vi "FPGAtdcControlTest.vi"() -> ()   [LabVIEW 2017]
uses:
  <vilib>/FPGAPlugInAG/PXI-7842R/niLvFpga_Open_PXI-7842R.vi
  <vilib>/rvi/interface/common/dynamic/niFpgaDynamicAddResources.vi
  <vilib>/rvi/interface/common/niFpgaWaitOnOcc.vi
  <vilib>/Utility/error.llb/Error Cluster From Error Code.vi
  <vilib>/rvi/errors/niLvFpgaAdjustHostInterfaceError.vi
  <vilib>/rvi/interface/nirviOpenFPGA/nirviOpenFPGA.xnode
  FPGA Bitfiles/Jarvis_FPGATargetMacro_281119simpleTDC_akCax+JGGYk.lvbitx
  <vilib>/rvi/interface/nirviMethod/nirviMethod.xnode
  <vilib>/rvi/interface/nirviReadWriteControl/nirviReadWriteControl.xnode
  NiFpgaLv.dll
  <vilib>/rvi/interface/Simulation/niFpgaSimulationCallBeginRW.vi
  <vilib>/rvi/errors/niLvFpgaMergeErrorWithErrorCode.vi
  <vilib>/FPGAPlugInAG/Dynamic/niLvFpga_ConfigureFifo_Dynamic.vi
  <vilib>/FPGAPlugInAG/Dynamic/niLvFpga_ReadFifo_Dynamic.vi
panel:
  out "error out":errorcluster
  out "Waveform Chart":u32[](graph)
  out "N acquired":i32
  out "Array":i32[](array[numeric])
  out "Histogram":dynamicdata(graph)
  out "tau":i16
  out "new data":bool
  in  "stop":bool
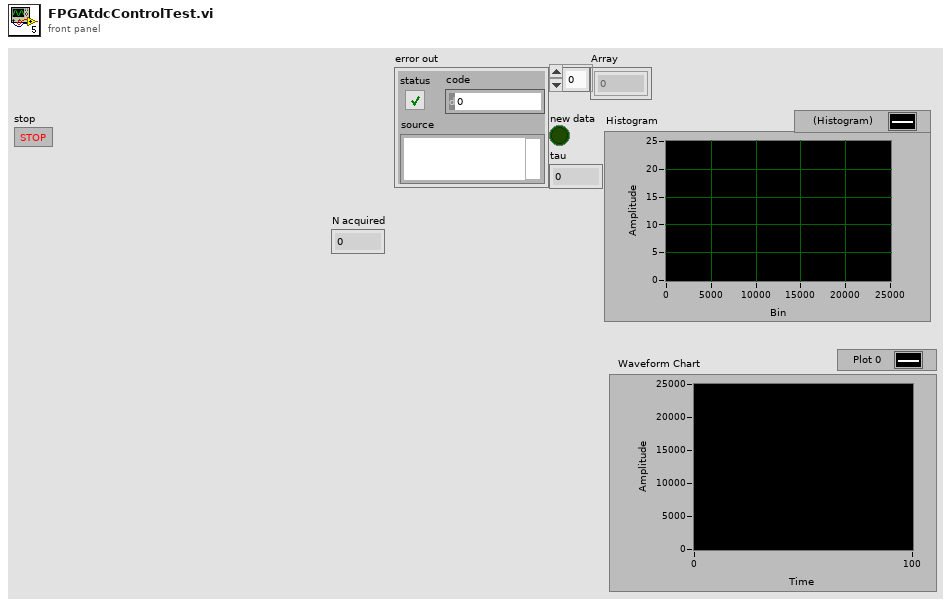
[diagram p1: front panel]
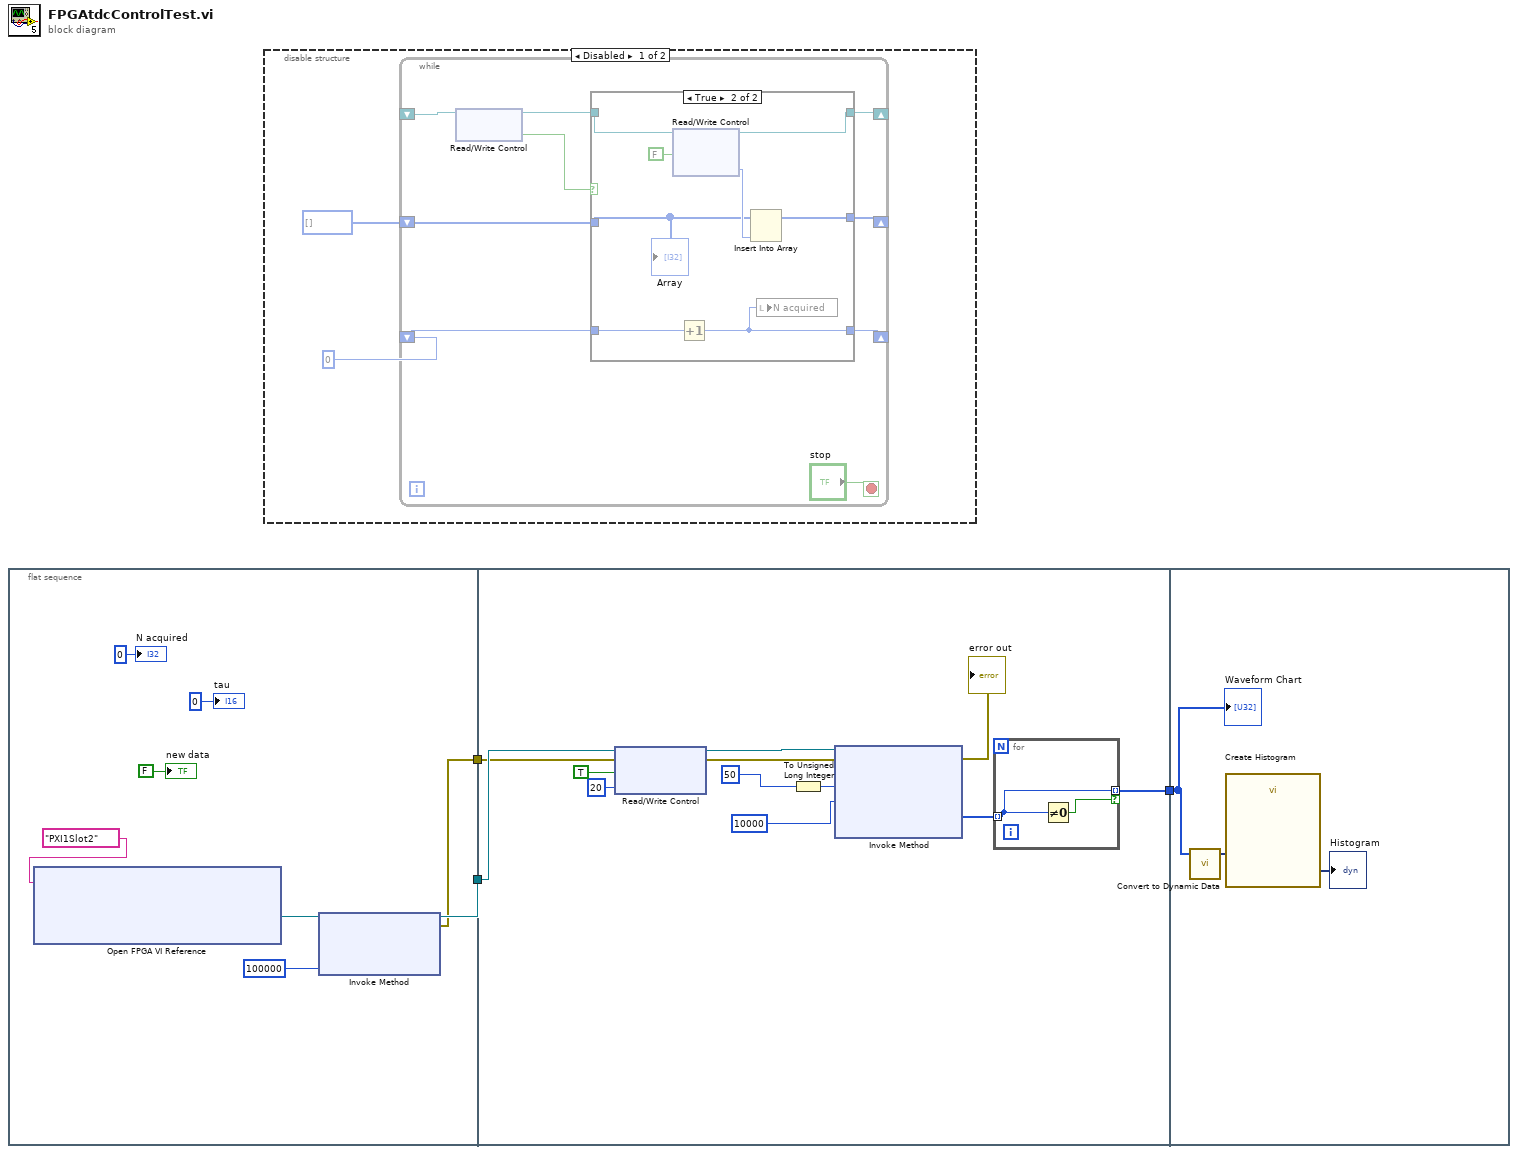
[diagram p0: block diagram]
diagram:
  n1 = flat-sequence {
    tunnel: [w5] -> w3
    tunnel: [w4] -> w1
    tunnel: w3 -> [w23]
    tunnel: [w16] -> w2
    tunnel: w1 -> [w14]
    tunnel: w2 -> [w26]
    frame #0 {
      n2 = xnode "Open FPGA VI Reference"("resource name"=tag "PXI1Slot2") -> ("FPGA VI Reference Out"=w7:refnum<k20>)  [unwired: 1 in, 1 out]
      n3 = xnode "Invoke Method"("FPGA VI Reference In"=w7, "Requested Depth"=u32 100000) -> ("FPGA VI Reference Out"=w5:refnum<k20>, "error out"=w4:errorcluster)  [unwired: 1 in, 1 out]
      "tau" <- i16 0 ("counts")
      "new data" <- FALSE ("Connector0/DIO5")
      "N acquired" <- 0 ("N acquired")
    }
    frame #1 {
      n4 = xnode "Read/Write Control"("FPGA VI Reference In"=w23, "error in"=w14, "Acquire times"=TRUE, "N photons"=u32 20) -> ("FPGA VI Reference Out"=w22:refnum<k20>, "error out"=w13:errorcluster)
      n5 = To Unsigned Long Integer(number=50) -> (unsigned 32bit integer=w19:u32)
      n6 = xnode "Invoke Method"("FPGA VI Reference In"=w22, "error in"=w13, "Number of Elements"=w19, "Timeout (ms)"=10000) -> ("error out"=→"error out":errorcluster, "Data"=w18:u32[])  [unwired: 2 out]
      n7 = for {
        tunnel: w18 -> [w25] mode=indexing
        tunnel: [w25] -> w16 mode=indexing if=w24
        n8 = Not Equal To 0?(x=w25) -> (x != 0?=w24:bool)
      }
    }
    frame #2 {
      n9 = call "Convert to Dynamic Data"("Array"=w26) -> ("Dynamic Data Type"=w27:dynamicdata)  [unwired: 3 in]
      n10 = call "Create Histogram"("Signal"=w27) -> ("Histogram"=→"Histogram":dynamicdata)  [unwired: 9 in, 1 out]
      "Waveform Chart" <- w26
    }
  }
  n11 = disable-structure shown="Disabled" {
    frame Disabled {
      n12 = while {
        shift-right: [w36] -> _
        shift-left: i32[] [] -> [w35]
        shift-right: [w34] -> _
        shift-left: [w39] -> w31
        shift-right: [w32] -> _
        shift-left: 0 ("N acquired") -> [w33]
        stop <- "stop" stop-if-true
        n13 = xnode "Read/Write Control"("FPGA VI Reference In"=w39) -> ("FPGA VI Reference Out"=w37:refnum<k20>, "new data"=w38:bool)  [unwired: 1 in, 1 out]
        n14 = case shown="True" w38 {
          tunnel: w35 -> [w43 w46]
          tunnel: w37 -> [w42 w51]
          tunnel: [w43 w48] -> w36
          tunnel: [w42 w47] -> w34
          tunnel: w33 -> [w41 w45]
          tunnel: [w41 w44] -> w32
          frame False {
          }
          frame True {
            n15 = xnode "Read/Write Control"("FPGA VI Reference In"=w51, "new data"=FALSE) -> ("FPGA VI Reference Out"=w47:refnum<k20>, "tau"=w49:i16)  [unwired: 1 in, 1 out]
            n16 = Increment(x=w45) -> (x+1=w44:i32)
            n17 = Insert Into Array(array=w46, new element=w49) -> (w48:i32[])  [unwired: 1 in]
            n18 = local write "N acquired"(w44) -> ()
            "Array" <- w46
          }
        }
      }
    }
    frame Enabled {
    }
  }
